vi "CT400_testwrap.vi"() -> ()   [LabVIEW 2009]
uses:
  CT400_lib.lvlib
panel:
  out "Error Init":i32
  in  "Laser Type":u32(ring) items=["LS_TunicsPlus", "LS_TunicsPurity", "LS_TunicsReference", "LS_TunicsT100s_HP", "LS_TunicsT100r", "LS_JdsuSws", "LS_Agilent", "NB_SOURCE"]
  out "CT400 Option":string
  out "# Spectral Lines":i32
  out "Spectral lines":dbl[](array[numeric]) format="%#.4f"
  in  "Resolution [pm]":u32 max=128 step=1
  out "#Nb of available \ndetectors":i32
  out "# Nb of available\ninputs":i32
  out "# of acquired points":i32
  out "Vext out":dbl format="%.4g"
  out "# of resampled points":i32
  out "Pout-interpolated":dbl[](array[numeric]) format="%.2g"
  out "Detector-interpolated":dbl[](array[numeric]) format="%.2g"
  out "Wavelength re-sampled":dbl[](array[numeric]) format="%.3g"
  in  "Interpolated data":string
  in  "Re-sampled wavelength":string
  in  "Detector data":string
  in  "Wavelength data":string
  out "Pout":dbl[](array[numeric]) format="%.2g"
  out "Detector":dbl[](array[numeric]) format="%#.2g"
  out "Wavelength":dbl[](array[numeric]) format="%.4f"
  out "P4 [dBm]":dbl format="%.2g"
  out "P3 [dBm]":dbl format="%.2g"
  out "P2 [dBm]":dbl format="%.2g"
  out "P1 [dBm]":dbl format="%.2g"
  out "Pout [dBm]":dbl format="%.2g"
  out "Error/warning":string
  out "error out":errorcluster
  in  "Start Wavelength [nm]":dbl
  in  "Laser power output [mW]":dbl
  in  "Stop Wavelength [nm]":dbl
  in  "Speed [nm/s]":i32
  in  "GPIB Address":i32
  in  "Upper Wavelength [nm]":dbl
  in  "Lower Wavelength [nm]":dbl
  in  "error in (no error)":errorcluster
  # "CT400 Settings"
  # "Data files (relative path)"
  # "Laser Settings"
  # "Power on detectors"
  # "Re-sampled Measurements"
  # "Measurements"
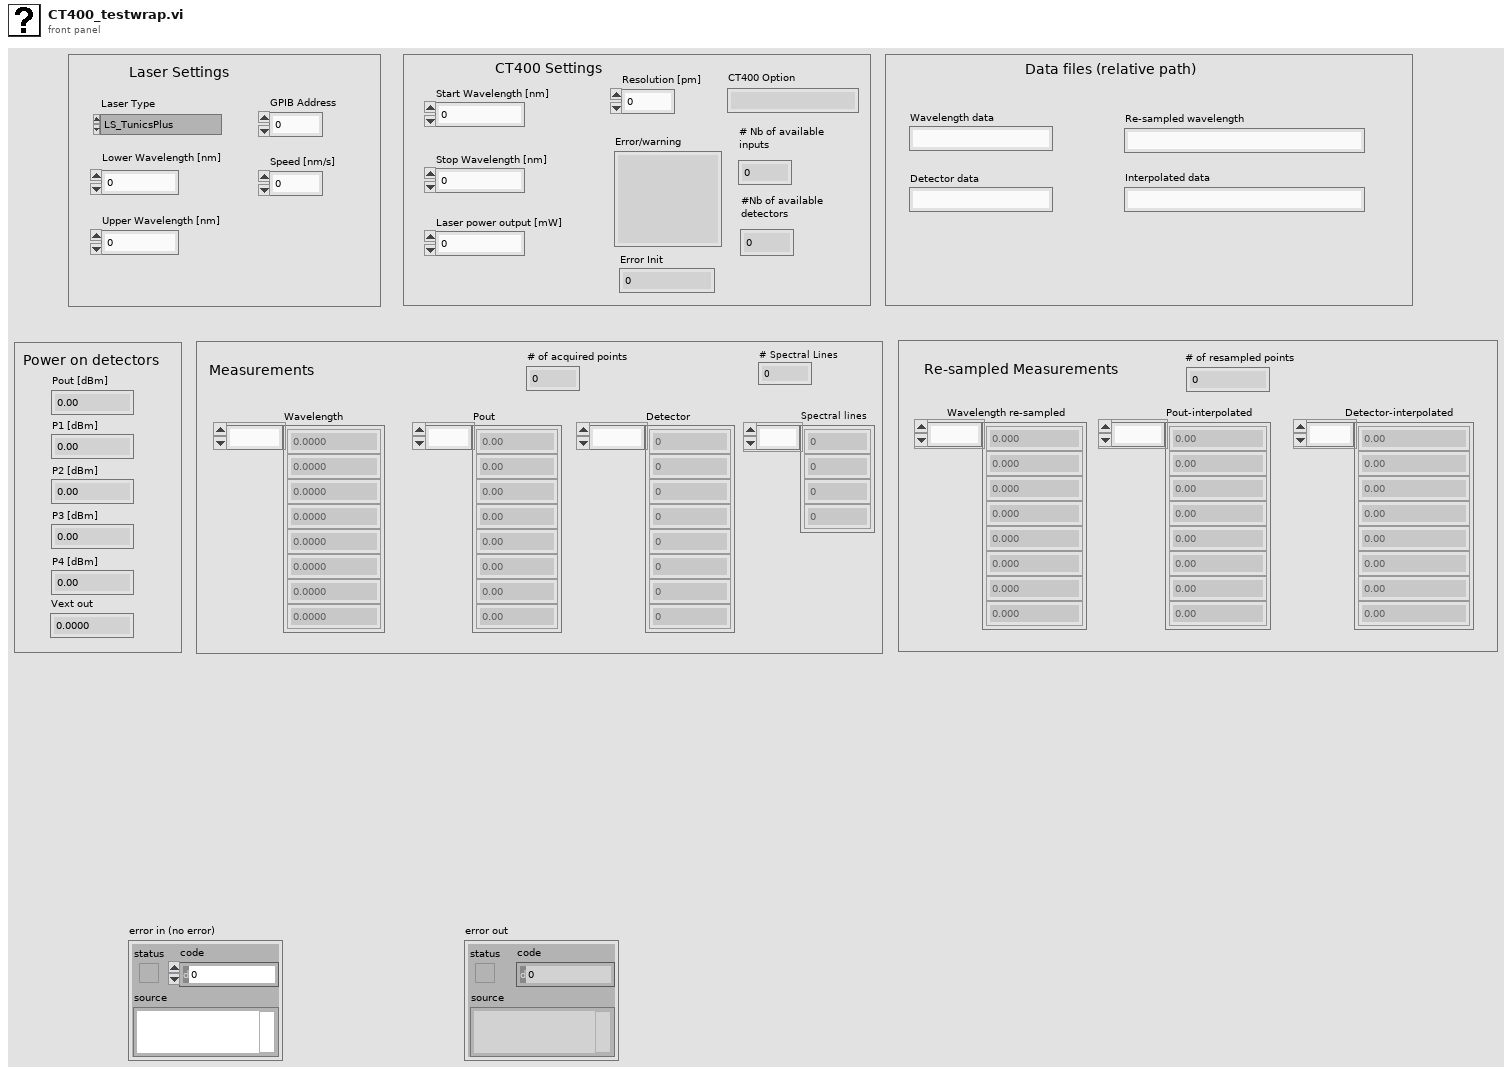
[diagram p1: front panel]
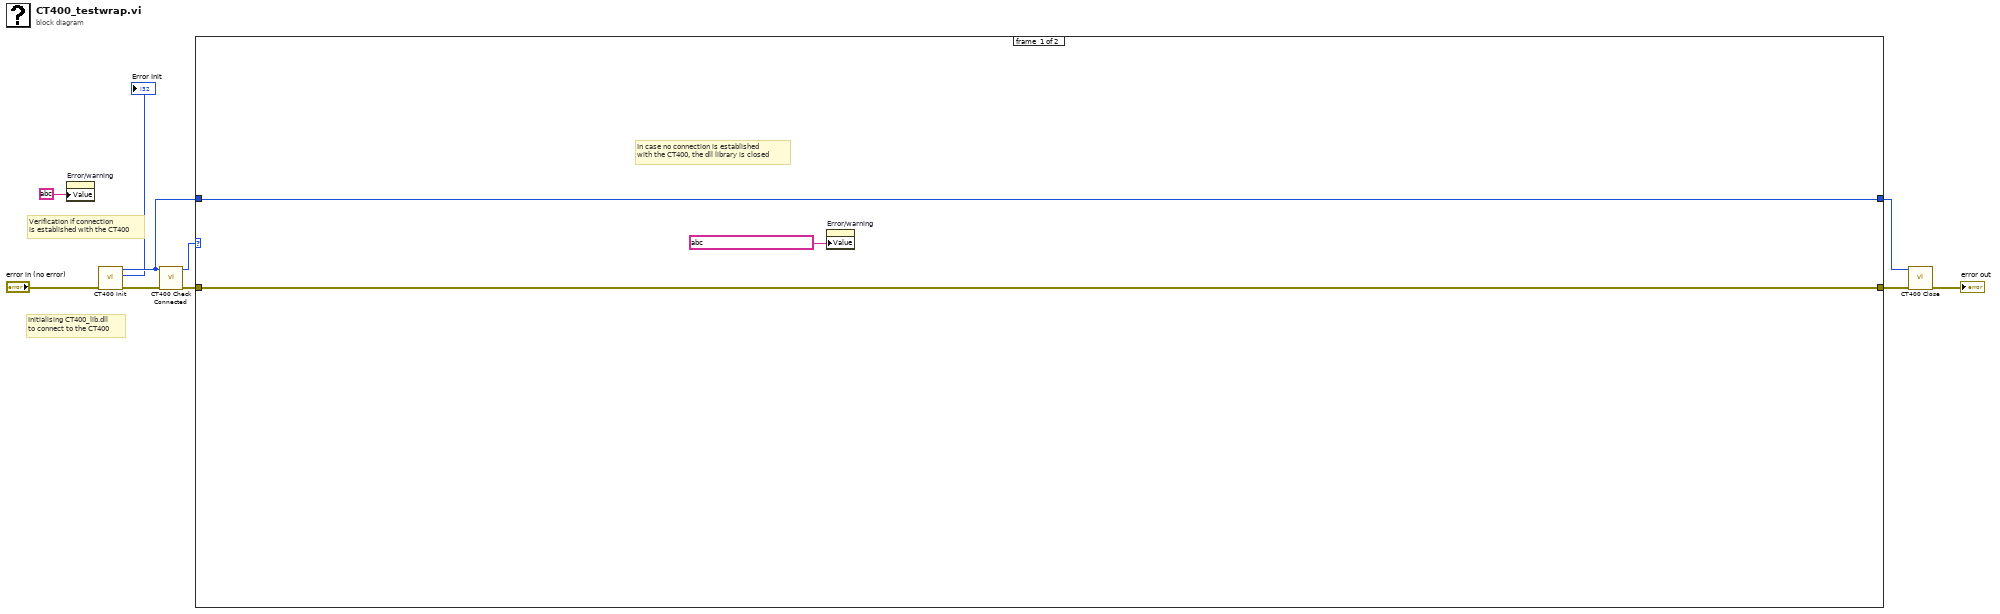
[diagram p0: block diagram]
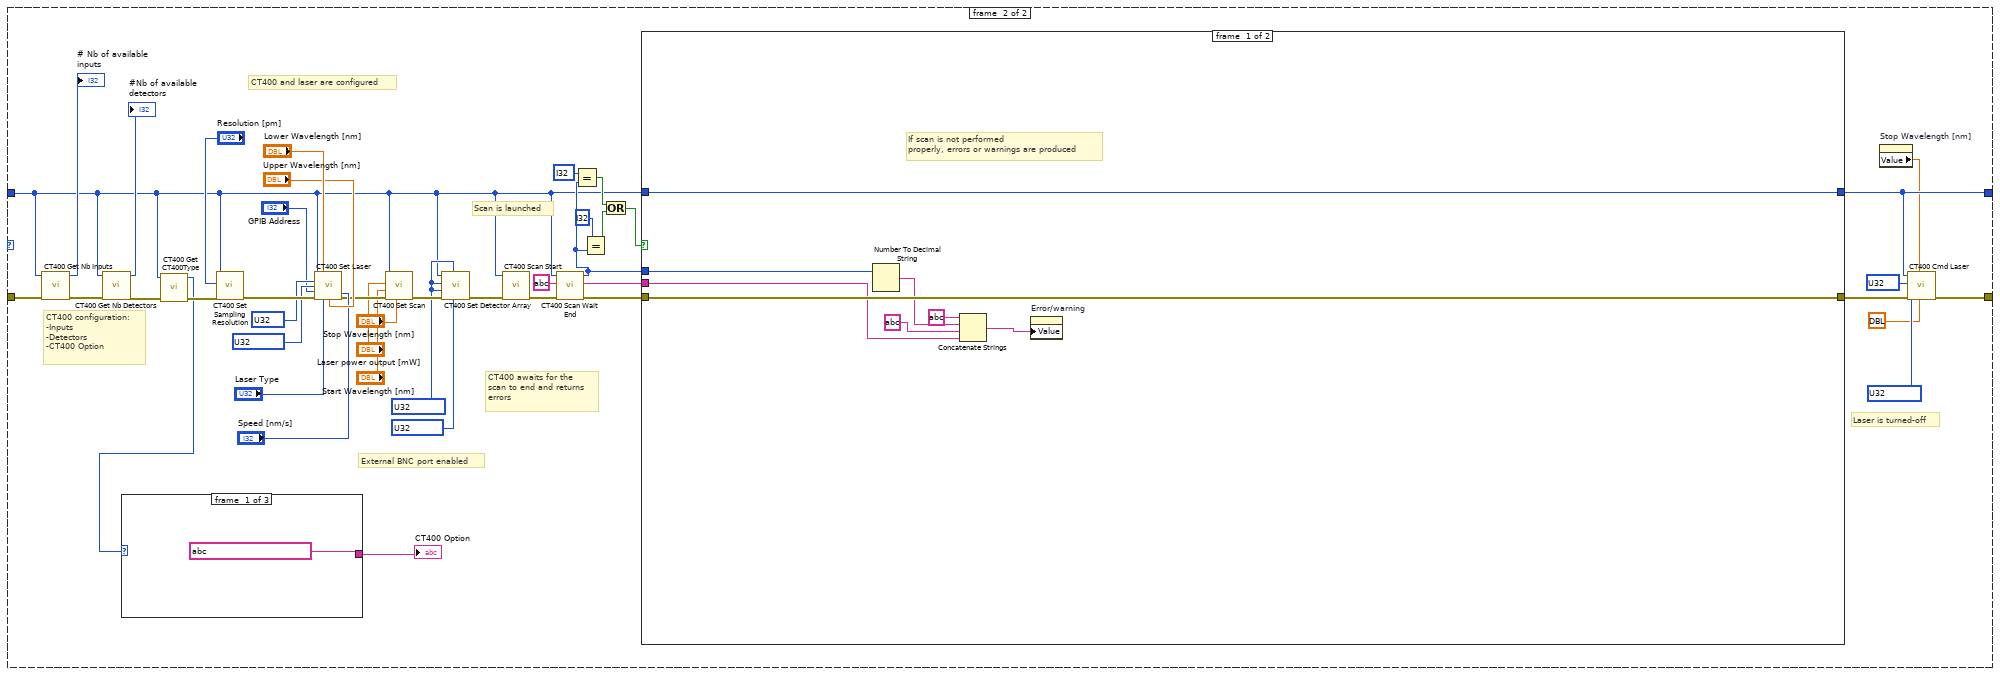
[diagram p2: hidden frame]
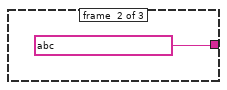
[diagram p3: hidden frame]
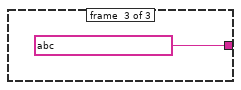
[diagram p4: hidden frame]
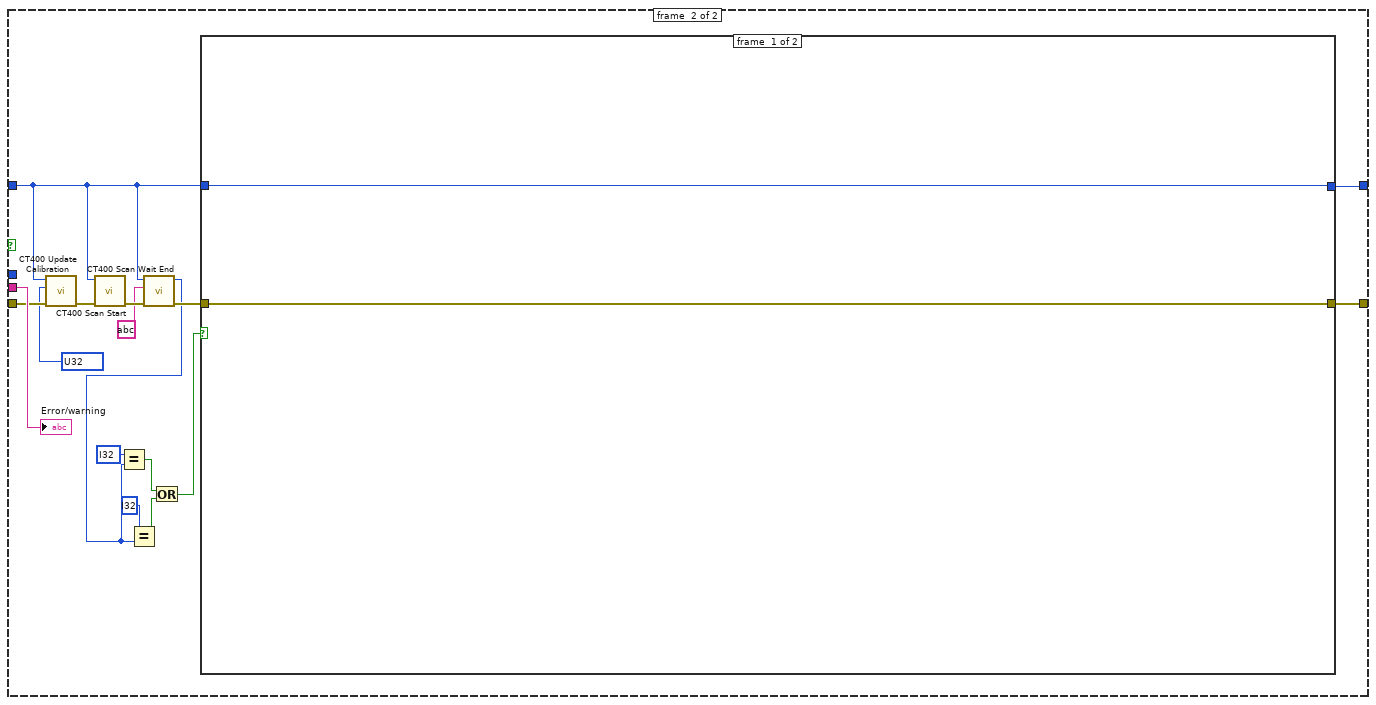
[diagram p5: hidden frame]
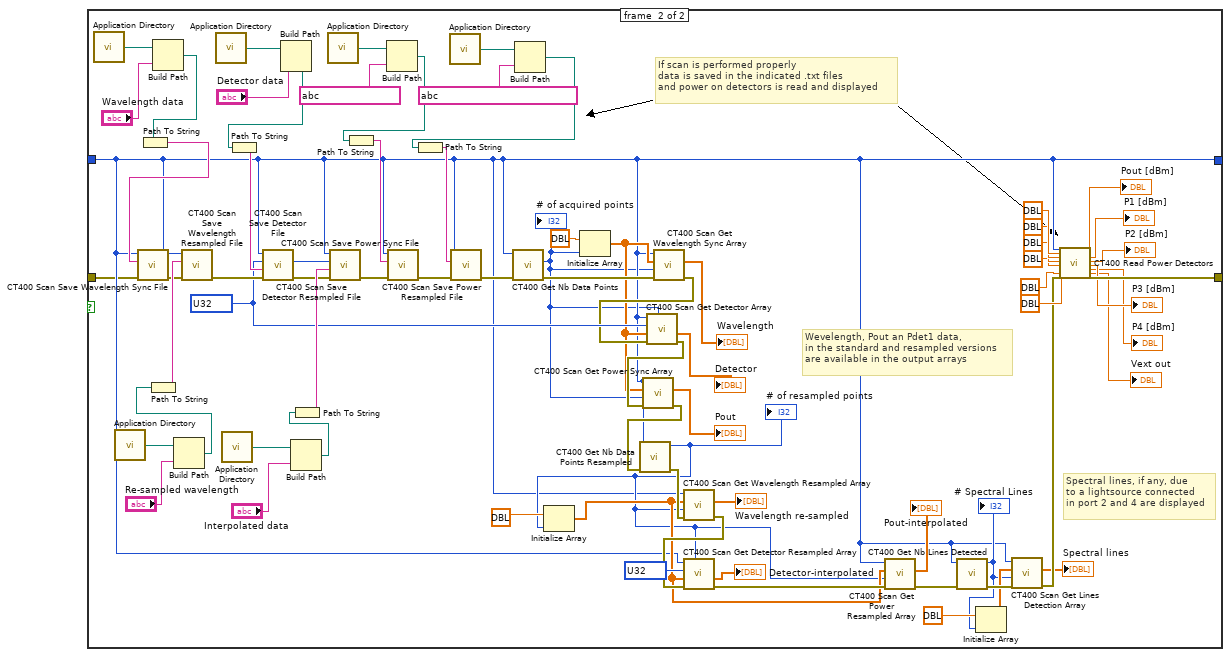
[diagram p6: hidden frame]
diagram:
  # "Verification if connection\nis established with the CT400"
  # "Initialising CT400_lib.dll\nto connect to the CT400"
  n1 = property on="Error/warning" class="Str"("Value"=string ?) -> ()  [unwired: 2 in, 2 out]
  n2 = call "CT400 Init.vi"("error in (no error)"="error in (no error)") -> ("error out"=w9:errorcluster, "iError out"=→"Error Init":i32, "function return"=w4:u64)  [unwired: 8 in]
  n3 = call "CT400 Check Connected.vi"("error in (no error)"=w9, "uiHandle"=w4) -> ("error out"=w7:errorcluster, "function return"=w8:i32)  [unwired: 8 in]
  n4 = case shown="1" w8 {
    tunnel: [w13 w41] -> w6
    tunnel: w7 -> [w13 w25]
    tunnel: [w12 w40] -> w5
    tunnel: w4 -> [w12 w18]
    frame #0 {
      # "In case no connection is established\nwith the CT400, the dll library is closed"
      n5 = property on="Error/warning" class="Str"("Value"=string ? ("Error/warning")) -> ()  [unwired: 2 in, 2 out]
    }
    frame #1 {
      w14 = u32 ? items=["DISABLE", "ENABLE"] ("eExt")
      w26 = u32 ? items=["DISABLE", "ENABLE"] ("eDect4")
      w38 = u32 ? items=["LI_1", "LI_2", "LI_3", "LI_4"] ("eLaser")
      w39 = u32 ? items=["DISABLE", "ENABLE"] ("eEnable")
      w54 = u32 ? items=["DISABLE", "ENABLE"] ("eEnable")
      w55 = u32 ? items=["LI_1", "LI_2", "LI_3", "LI_4"] ("eLaser")
      # "CT400 configuration:\n-Inputs\n-Detectors\n-CT400 Option"
      # "External BNC port enabled"
      # "Laser is turned-off"
      # "CT400 awaits for the\nscan to end and returns\nerrors"
      # "Scan is launched"
      # "CT400 and laser are configured"
      n6 = call "CT400 Get Nb Inputs.vi"("error in (no error)"=w25, "uiHandle"=w18) -> ("error out"=w23:errorcluster, "function return"=→"# Nb of available\ninputs":i32)  [unwired: 8 in]
      n7 = call "CT400 Get Nb Detectors.vi"("error in (no error)"=w23, "uiHandle"=w18) -> ("error out"=w19:errorcluster, "function return"=→"#Nb of available \ndetectors":i32)  [unwired: 8 in]
      n8 = call "CT400 Get CT400Type.vi"("error in (no error)"=w19, "uiHandle"=w18) -> ("error out"=w20:errorcluster, "function return"=w17:i32)  [unwired: 8 in]
      n9 = case shown="2" w17 {
        tunnel: [string ? ("CT400 Option") string ? ("CT400 Option") string ? ("CT400 Option")] -> w16
        frame #0 {
        }
        frame #1 {
        }
        frame #2 {
        }
      }
      "CT400 Option" <- w16
      n10 = call "CT400 Set Sampling Resolution.vi"("error in (no error)"=w20, "uiResolution"="Resolution [pm]", "uiHandle"=w18) -> ("error out"=w56:errorcluster)  [unwired: 7 in, 1 out]
      n11 = call "CT400 Set Laser.vi"("uiHandle"=w18, "eLaserType"="Laser Type", "dMaxWavelength"="Upper Wavelength [nm]", "eLaser"=w55, "eEnable"=w54, "iGPIBAdress"="GPIB Address", "error in (no error)"=w56, "dMinWavelength"="Lower Wavelength [nm]", "Speed"="Speed [nm/s]") -> ("error out"=w49:errorcluster)  [unwired: 5 in, 1 out]
      n12 = call "CT400 Set Scan.vi"("dMaxWavelength"="Stop Wavelength [nm]", "error in (no error)"=w49, "dMinWavelength"="Start Wavelength [nm]", "dLaserPower"="Laser power output [mW]", "uiHandle"=w18) -> ("error out"=w28:errorcluster)  [unwired: 5 in, 1 out]
      n13 = call "CT400 Set Detector Array.vi"("eExt"=w14, "eDect4"=w26, "error in (no error)"=w28, "eDect3"=w26, "eDect2"=w26, "uiHandle"=w18) -> ("error out"=w27:errorcluster)  [unwired: 4 in, 1 out]
      n14 = call "CT400 Scan Start.vi"("error in (no error)"=w27, "uiHandle"=w18) -> ("error out"=w29:errorcluster)  [unwired: 8 in, 1 out]
      n15 = call "CT400 Scan Wait End.vi"("error in (no error)"=w29, "tcError"=string ?, "uiHandle"=w18) -> ("error out"=w44:errorcluster, "tcError out"=w43:string, "function return"=w34:i32)  [unwired: 6 in]
      n16 = Equal?(x=i32 ?, y=w34) -> (x = y?=w31:bool)
      n17 = Equal?(x=i32 ?, y=w34) -> (x = y?=w32:bool)
      n18 = Or(x=w31, y=w32) -> (x .or. y?=w30:bool)
      n19 = case shown="True" w30 {
        tunnel: [w67 w82] -> w42
        tunnel: w18 -> [w66 w77]
        tunnel: w44 -> [w67 w81]
        tunnel: w43 -> [w63 w83]
        tunnel: [w66 w76] -> w40
        tunnel: w34 -> [w65 _]
        frame #0 {
          # "If scan is not performed \nproperly, errors or warnings are produced"
          n20 = Number To Decimal String(number=w65) -> (decimal integer string=w64:string)  [unwired: 1 in]
          n21 = Concatenate Strings(string ? ("string"), w64, string ? ("string"), w63) -> (w62:string)
          n22 = property on="Error/warning" class="Str"("Value"=w62) -> ()  [unwired: 2 in, 2 out]
        }
        frame #1 {
          w80 = u32 ? items=["DE_1", "DE_2", "DE_3", "DE_4", "DE_5"] ("eDetector")
          n23 = call "CT400 Update Calibration.vi"("error in (no error)"=w81, "eDetector"=w80, "uiHandle"=w77) -> ("error out"=w79:errorcluster)  [unwired: 7 in, 1 out]
          n24 = call "CT400 Scan Start.vi"("error in (no error)"=w79, "uiHandle"=w77) -> ("error out"=w78:errorcluster)  [unwired: 8 in, 1 out]
          n25 = call "CT400 Scan Wait End.vi"("error in (no error)"=w78, "tcError"=string ?, "uiHandle"=w77) -> ("error out"=w75:errorcluster, "function return"=w69:i32)  [unwired: 6 in, 1 out]
          n26 = Equal?(x=i32 ?, y=w69) -> (x = y?=w73:bool)
          n27 = Equal?(x=i32 ?, y=w69) -> (x = y?=w72:bool)
          n28 = Or(x=w73, y=w72) -> (x .or. y?=w68:bool)
          n29 = case shown="True" w68 {
            tunnel: [w84 w156] -> w82
            tunnel: w77 -> [w85 w88]
            tunnel: [w85 w88] -> w76
            tunnel: w75 -> [w84 w87]
            frame #0 {
            }
            frame #1 {
              w125 = u32 ? items=["DE_1", "DE_2", "DE_3", "DE_4", "DE_5"] ("eDetector")
              w128 = u32 ? items=["DE_1", "DE_2", "DE_3", "DE_4"] ("Detector")
              # "Spectral lines, if any, due\nto a lightsource connected\nin port 2 and 4 are displayed"
              # "Wevelength, Pout an Pdet1 data,\nin the standard and resampled versions\nare available in the output arrays"
              # "If scan is performed properly\ndata is saved in the indicated .txt files\nand power on detectors is read and displayed"
              n30 = call <vilib>:"Application Directory.vi"() -> ("Application Directory"=w89:path)
              n31 = call <vilib>:"Application Directory.vi"() -> ("Application Directory"=w139:path)
              n32 = Build Path(base path=w89, name or relative path="Wavelength data") -> (appended path=w143:path)
              n33 = Path To String(path=w143) -> (string=w158:string)
              n34 = call "CT400 Scan Save Wavelength Sync File.vi"("error in (no error)"=w87, "pcPath"=w158, "uiHandle"=w88) -> ("error out"=w135:errorcluster)  [unwired: 6 in, 2 out]
              n35 = Build Path(base path=w139, name or relative path="Re-sampled wavelength") -> (appended path=w137:path)
              n36 = Path To String(path=w137) -> (string=w136:string)
              n37 = call "CT400 Scan Save Wavelength Resampled File.vi"("error in (no error)"=w135, "pcPath"=w136, "uiHandle"=w88) -> ("error out"=w134:errorcluster)  [unwired: 6 in, 2 out]
              n38 = call <vilib>:"Application Directory.vi"() -> ("Application Directory"=w142:path)
              n39 = call <vilib>:"Application Directory.vi"() -> ("Application Directory"=w133:path)
              n40 = Build Path(base path=w142, name or relative path="Detector data") -> (appended path=w140:path)
              n41 = Path To String(path=w140) -> (string=w157:string)
              n42 = call "CT400 Scan Save Detector File.vi"("error in (no error)"=w134, "pcPath"=w157, "eDetector"=w128, "uiHandle"=w88) -> ("error out"=w129:errorcluster)  [unwired: 5 in, 2 out]
              n43 = Build Path(base path=w133, name or relative path="Interpolated data") -> (appended path=w131:path)
              n44 = Path To String(path=w131) -> (string=w130:string)
              n45 = call <vilib>:"Application Directory.vi"() -> ("Application Directory"=w111:path)
              n46 = call "CT400 Scan Save Detector Resampled File.vi"("error in (no error)"=w129, "pcPath"=w130, "eDetector"=w128, "uiHandle"=w88) -> ("error out"=w117:errorcluster)  [unwired: 5 in, 2 out]
              n47 = Build Path(base path=w111, name or relative path=string ?) -> (appended path=w112:path)
              n48 = Path To String(path=w112) -> (string=w108:string)
              n49 = call "CT400 Scan Save Power Sync File.vi"("error in (no error)"=w117, "pcPath"=w108, "uiHandle"=w88) -> ("error out"=w116:errorcluster)  [unwired: 6 in, 2 out]
              n50 = call <vilib>:"Application Directory.vi"() -> ("Application Directory"=w113:path)
              n51 = Build Path(base path=w113, name or relative path=string ?) -> (appended path=w114:path)
              n52 = Path To String(path=w114) -> (string=w107:string)
              n53 = call "CT400 Scan Save Power Resampled File.vi"("error in (no error)"=w116, "pcPath"=w107, "uiHandle"=w88) -> ("error out"=w115:errorcluster)  [unwired: 6 in, 2 out]
              n54 = call "CT400 Get Nb Data Points.vi"("error in (no error)"=w115, "uiHandle"=w88) -> ("error out"=w119:errorcluster, "iDataPoints out"=w86:i32)  [unwired: 6 in, 2 out]
              "# of acquired points" <- w86
              n55 = Initialize Array(dbl ? ("element"), w86) -> (w103:dbl[])
              n56 = call "CT400 Scan Get Wavelength Sync Array.vi"("error in (no error)"=w119, "iArraySize"=w86, "dArray"=w103, "uiHandle"=w88) -> ("error out"=w118:errorcluster, "dArray out"=→"Wavelength":dbl[])  [unwired: 5 in, 1 out]
              n57 = call "CT400 Scan Get Detector Array.vi"("iArraySize"=w86, "error in (no error)"=w118, "dArray"=w103, "eDetector"=w128, "uiHandle"=w88) -> ("error out"=w145:errorcluster, "dArray out"=→"Detector":dbl[])  [unwired: 4 in, 1 out]
              n58 = call "CT400 Scan Get Power Sync Array.vi"("error in (no error)"=w145, "iArraySize"=w86, "dArray"=w103, "uiHandle"=w88) -> ("error out"=w102:errorcluster, "dArray out"=→"Pout":dbl[])  [unwired: 5 in, 1 out]
              n59 = call "CT400 Get Nb Data Points Resampled.vi"("error in (no error)"=w102, "uiHandle"=w88) -> ("error out"=w101:errorcluster, "function return"=w98:i32)  [unwired: 8 in]
              "# of resampled points" <- w98
              n60 = Initialize Array(dbl ? ("element"), w98) -> (w100:dbl[])
              n61 = call "CT400 Scan Get Wavelength Resampled Array.vi"("error in (no error)"=w101, "iArraySize"=w98, "dArray"=w100, "uiHandle"=w88) -> ("error out"=w127:errorcluster, "dArray out"=→"Wavelength re-sampled":dbl[])  [unwired: 5 in, 1 out]
              n62 = call "CT400 Scan Get Detector Resampled Array.vi"("iArraySize"=w98, "error in (no error)"=w127, "dArray"=w100, "eDetector"=w125, "uiHandle"=w88) -> ("error out"=w126:errorcluster, "dArray out"=→"Detector-interpolated":dbl[])  [unwired: 4 in, 1 out]
              n63 = call "CT400 Scan Get Power Resampled Array.vi"("error in (no error)"=w126, "iArraySize"=w98, "dArray"=w100, "uiHandle"=w88) -> ("error out"=w97:errorcluster, "dArray out"=→"Pout-interpolated":dbl[])  [unwired: 5 in, 1 out]
              n64 = call "CT400 Get Nb Lines Detected.vi"("error in (no error)"=w97, "uiHandle"=w88) -> ("error out"=w96:errorcluster, "function return"=w93:i32)  [unwired: 8 in]
              "# Spectral Lines" <- w93
              n65 = Initialize Array(dbl ? ("element"), w93) -> (w94:dbl[])
              n66 = call "CT400 Scan Get Lines Detection Array.vi"("error in (no error)"=w96, "iArraySize"=w93, "dArray"=w94, "uiHandle"=w88) -> ("error out"=w92:errorcluster, "dArray out"=→"Spectral lines":dbl[])  [unwired: 5 in, 1 out]
              n67 = call "CT400 Read Power Detectors.vi"("uiHandle"=w88, "Pout"=dbl ?, "P1"=dbl ?, "P2"=dbl ?, "P3"=dbl ?, "P4"=dbl ?, "Vext"=dbl ?, "error in (no error)"=w92) -> ("Pout out"=→"Pout [dBm]":dbl, "P1 out"=→"P1 [dBm]":dbl, "P2 out"=→"P2 [dBm]":dbl, "P3 out"=→"P3 [dBm]":dbl, "P4 out"=→"P4 [dBm]":dbl, "Vext out"=→"Vext out":dbl, "error out"=w156:errorcluster)  [unwired: 12 in, 1 out]
            }
          }
          "Error/warning" <- w83
        }
      }
      n68 = property on="Stop Wavelength [nm]" class="DigNum (strict)"() -> ("Value"=w36:dbl)  [unwired: 2 in, 2 out]
      n69 = call "CT400 Cmd Laser.vi"("dPower"=dbl ?, "dWavelength"=w36, "error in (no error)"=w42, "eEnable"=w39, "eLaser"=w38, "uiHandle"=w40) -> ("error out"=w41:errorcluster)  [unwired: 4 in, 1 out]
    }
  }
  n70 = call "CT400 Close.vi"("error in (no error)"=w6, "uiHandle"=w5) -> ("error out"=→"error out":errorcluster)  [unwired: 8 in, 1 out]
